vi "Save Vibration Config.vi"(8 "error in (no error)":errorcluster, 10 "Accell Config":T1 {"PS Cutoff Frequency"."HP Passband" min=1.0 step=1.0 format="%#.4f"; "PS Cutoff Frequency"."LP Stopband" min=1.0 step=1.0 format="%#.4f"; "PS Cutoff Frequency"."HP Stopband" min=1.0 step=1.0 format="%#.4f"; "PS Cutoff Frequency"."LP Passband" min=1.0 step=1.0 format="%#.4f"; "GB Cutoff Frequency"."HP Passband" min=1.0 step=1.0 format="%#.4f"; "GB Cutoff Frequency"."LP Stopband" min=1.0 step=1.0 format="%#.4f"; "GB Cutoff Frequency"."HP Stopband" min=1.0 step=1.0 format="%#.4f"; "GB Cutoff Frequency"."LP Passband" min=1.0 step=1.0 format="%#.4f"; "Fan Cutoff Frequency"."HP Passband" min=1.0 step=1.0 format="%#.4f"; "Fan Cutoff Frequency"."LP Stopband" min=1.0 step=1.0 format="%#.4f"; "Fan Cutoff Frequency"."HP Stopband" min=1.0 step=1.0 format="%#.4f"; "Fan Cutoff Frequency"."LP Passband" min=1.0 step=1.0 format="%#.4f"}, 11 "Path":path) -> (0 "error out":errorcluster)   [LabVIEW 2018, in "File IO.lvlib"]
uses:
  File IO.lvlib
  Testing UI 3/Public Controls/Accel Config.ctl
  Testing UI 3/Private Controls/Cutoff Frequency.ctl
  <vilib>/Utility/NIReport.llb/Report Type.ctl
  <vilib>/Utility/NIReport.llb/NI_report.lvclass
  <vilib>/addons/_office/NI_ReportGenerationToolkit.lvlib
  <vilib>/Utility/NIReport.llb/NI_ReportGenerationCore.lvlib
  <vilib>/Utility/NIReport.llb/Excel/NI_Excel.lvclass
  Testing UI 3/Testing UI 3.lvlib
panel:
  # "Highpass Cutoff Frequency"
  # "Lowpass Cutoff Frequency"
  # "Highpass Cutoff Frequency"
  # "Lowpass Cutoff Frequency"
  # "Highpass Cutoff Frequency"
  # "Lowpass Cutoff Frequency"
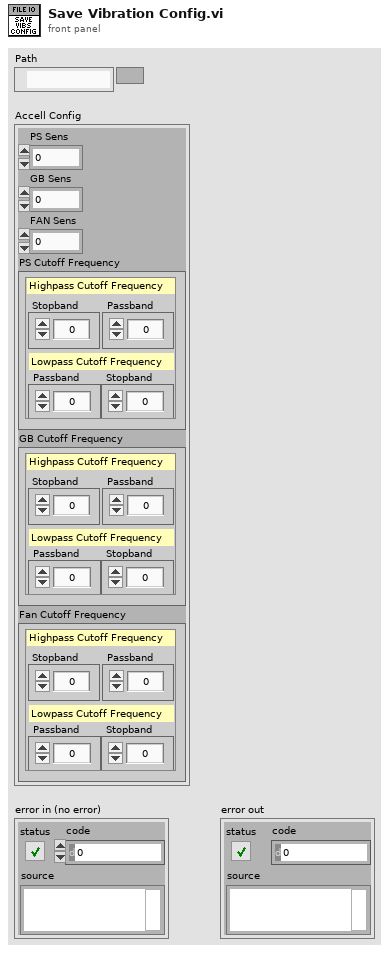
[diagram p1: front panel]
types:
  T1 = typedef "Testing UI 3.lvlib/Accel Config.ctl" = cluster{"PS Sens":dbl, "GB Sens":dbl, "FAN Sens":dbl, "PS Cutoff Frequency":T2, "GB Cutoff Frequency":T2, "Fan Cutoff Frequency":T2}
  T2 = typedef "Testing UI 3.lvlib/Cutoff Frequency.ctl" = cluster{"LP Passband":dbl, "HP Stopband":dbl, "LP Stopband":dbl, "HP Passband":dbl}
  T3 = typedef "NI_ReportGenerationCore.lvlib/Report Type.ctl" = enum16{"HTML", "Word", "Excel"}
  T4 = enum16{"maximized", "minimized", "normal", "no change"}
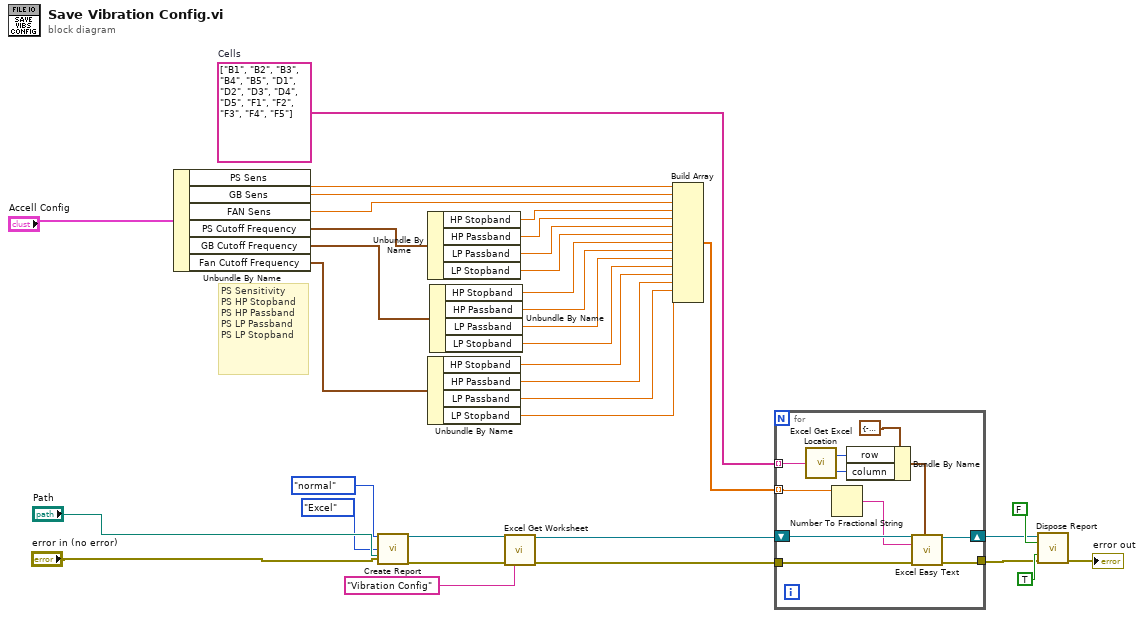
[diagram p0: block diagram]
diagram:
  w32 = string[] ["B1", "B2", "B3", "B4", "B5", "D1", "D2", "D3", "D4", "D5", "F1", "F2", "F3", "F4", "F5"]  # Cells
  # "PS Sensitivity\nPS HP Stopband\nPS HP Passband\nPS LP Passband\nPS LP Stopband"
  n1 = Unbundle By Name("Accell Config") -> ("PS Sens"=w16:dbl, "GB Sens"=w17:dbl, "FAN Sens"=w18:dbl, "PS Cutoff Frequency"=w13:T2, "GB Cutoff Frequency"=w14:T2, "Fan Cutoff Frequency"=w15:T2)
  n2 = call <vilib>:"Create Report.vi"("window state (normal)"=T4."normal", "report type"=Report_Type."Excel", "template (empty)"="Path", "error in (no error)"="error in (no error)") -> ("report out"=w3:refnum<class "NI_report.lvclass">, "error out"=w4:errorcluster)  [unwired: 10 in]
  n3 = Unbundle By Name(w13) -> ("HP Stopband"=w19:dbl, "HP Passband"=w20:dbl, "LP Passband"=w21:dbl, "LP Stopband"=w22:dbl)
  n4 = Unbundle By Name(w15) -> ("HP Stopband"=w27:dbl, "HP Passband"=w28:dbl, "LP Passband"=w29:dbl, "LP Stopband"=w30:dbl)
  n5 = Unbundle By Name(w14) -> ("HP Stopband"=w23:dbl, "HP Passband"=w24:dbl, "LP Passband"=w25:dbl, "LP Stopband"=w26:dbl)
  n6 = call <vilib>:"Excel Get Worksheet.vi"("report in"=w3, "error in (no error)"=w4, "name (\"\")"="Vibration Config" ("name (\"\")")) -> ("report out"=w9:refnum<class "NI_report.lvclass">, "error out"=w10:errorcluster)  [unwired: 11 in]
  n7 = Build Array(w16, w17, w18, w19, w20, w21, w22, w23, w24, w25, w26, w27, w28, w29, w30) -> (w31:dbl[])
  n8 = for {
    shift-right: [w43] -> w5
    shift-left: w9 -> [w44]
    tunnel: [w45] -> w6
    tunnel: w10 -> [w46]
    tunnel: w31 -> [w37] mode=indexing
    tunnel: w32 -> [w36] mode=indexing
    n9 = call <vilib>:"Excel Get Excel Location.vi"("cell's name"=w36) -> ("row"=w39:i32, "column"=w38:i32)
    n10 = Number To Fractional String(number=w37) -> (F-format string=w40:string)  [unwired: 3 in]
    n11 = Bundle By Name(cluster=cluster{"row":i32, "column":i32} {"row"=-1, "column"=-1} ("start (-1, -1)"), "row"=w39, "column"=w38) -> (w41:cluster{"row":i32, "column":i32})
    n12 = call <vilib>:"Excel Easy Text.vi"("report in"=w44, "text"=w40, "start (-1, -1)"=w41, "end (-1, -1)"=w41, "error in (no error)"=w46) -> ("report out"=w43:refnum<class "NI_report.lvclass">, "error out"=w45:errorcluster)  [unwired: 6 in, 3 out]
  }
  n13 = call-dynamic "Dispose Report.vi"("report in"=w5, "wait until printing completed? (T)"=FALSE, "save changes? (F)"=TRUE, "error in (no error)"=w6) -> ("error out"=→"error out":errorcluster)  [unwired: 11 in]
